vi "solar_app Resolve Path.vi"(0 "Path to Resolve (\"\"=default Path)":string, 1 "default Path":path) -> (5 "Is Relative Path?":bool, 6 "Resolved Path":path)   [LabVIEW 2018]
doc: "This resolves the relative or absolute path."
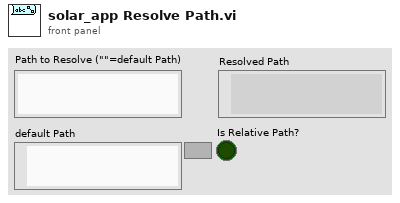
[diagram p1: front panel]
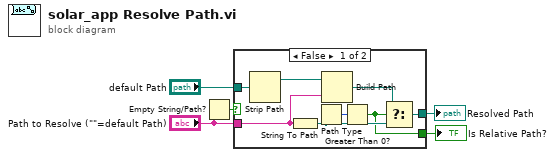
[diagram p0: block diagram]
diagram:
  n1 = Empty String/Path?(string/path="Path to Resolve (\"\"=default Path)") -> (empty?=w5:bool)
  n2 = case shown="False" w5 {
    tunnel: "Path to Resolve (\"\"=default Path)" -> [w10 _]
    tunnel: "default Path" -> [w13 w14]
    tunnel: [w8 w14] -> w2
    tunnel: [w6 _] -> w1
    frame False {
      n3 = Strip Path(path=w13) -> (stripped path=w7:path)  [unwired: 1 out]
      n4 = String To Path(string=w10) -> (path=w9:path)
      n5 = Path Type(1:w9) -> (0:w12:i16)
      n6 = Build Path(base path=w7, name or relative path=w10) -> (appended path=w11:path)
      n7 = Greater Than 0?(x=w12) -> (x > 0?=w6:bool)
      n8 = Select(t=w11, s=w6, f=w9) -> (s? t:f=w8:path)
    }
    frame True {
    }
  }
  "Resolved Path" <- w2
  "Is Relative Path?" <- w1
